vi "Function.vi"(8 "error in (no error)":errorcluster, 9 "Numeric B":T1, 10 "Numeric A":T1, 11 "Two Terminal in":refnum<class "Add_CPLX_EXT.lvclass">) -> (0 "error out":errorcluster, 2 "Result":T1, 3 "Two Terminal out":refnum<class "Add_CPLX_EXT.lvclass">)   [LabVIEW 2021, in "Add_CPLX_EXT.lvclass"]
uses:
  Add_CPLX_EXT.lvclass
  Type.ctl
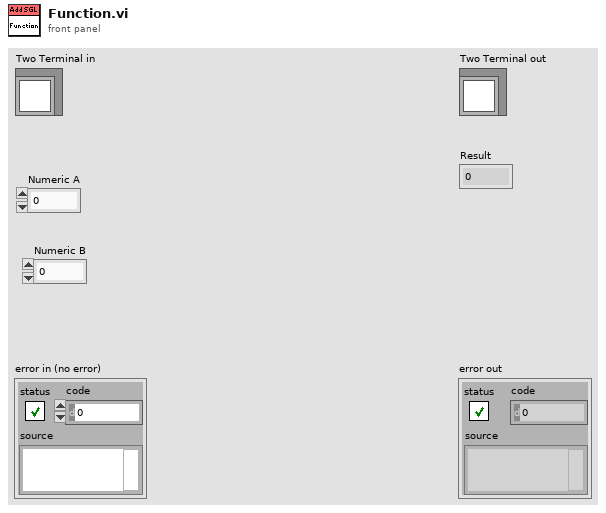
[diagram p1: front panel]
types:
  T1 = typedef "Add_CPLX_EXT.lvclass/Type.ctl" = cxt
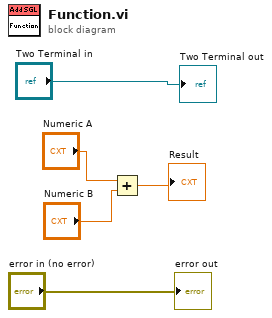
[diagram p0: block diagram]
diagram:
  n1 = Add(x="Numeric A", y="Numeric B") -> (x+y=→"Result":T1)
  "error out" <- "error in (no error)"
  "Two Terminal out" <- "Two Terminal in"
